vi "Read Max acceleration.vi"(8 "error in (no error)":errorcluster, 11 "Motor-Maxon in":refnum<class "Motor-Maxon.lvclass">) -> (0 "error out":errorcluster, 2 "Max acceleration":dbl caption="Max. acceleration [rpm/sec]", 3 "Motor-Maxon out":refnum<class "Motor-Maxon.lvclass">)   [LabVIEW 2013, in "PowderDeposition.lvlib" / "Motor-Maxon.lvclass"]
uses:
  Motor-Maxon.lvclass
  Motor-Maxon.lvclass/Motor-Maxon.ctl
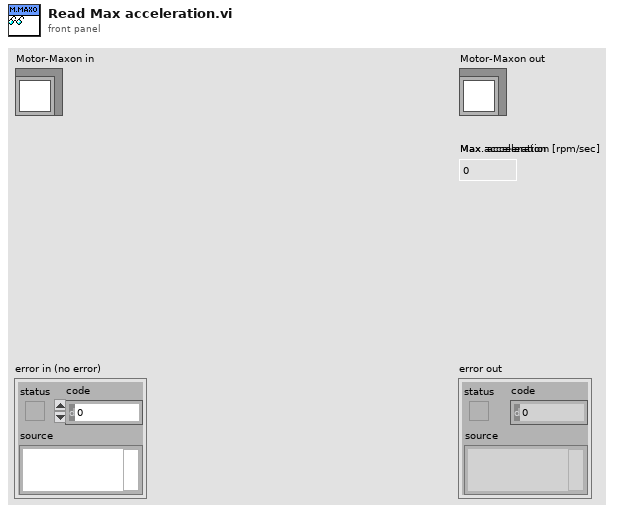
[diagram p1: front panel]
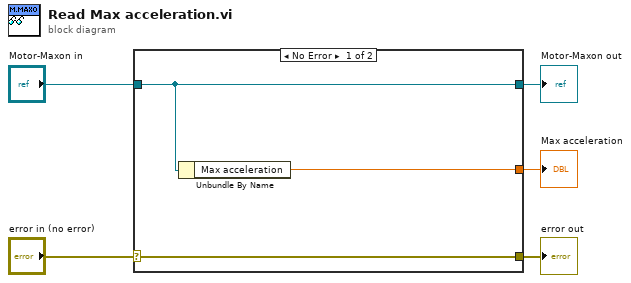
[diagram p0: block diagram]
diagram:
  n1 = case shown="No Error" "error in (no error)" {
    selector: "error in (no error)" -> [w8 w9]
    tunnel: [w8 w9] -> w4
    tunnel: [w7 w10] -> w2
    tunnel: "Motor-Maxon in" -> [w7 w10]
    tunnel: [w6 _] -> w1
    frame No Error {
      n2 = Unbundle By Name(w7) -> ("Max acceleration"=w6:dbl)
    }
    frame Error {
    }
  }
  "error out" <- w4
  "Motor-Maxon out" <- w2
  "Max acceleration" <- w1
